vi "Ka-THWAP grabbers.vi"(10 "Action":enum16{"None", "Left", "Right", "Yes"}(ring), 11 "Enum":T1) -> ()   [LabVIEW 2014]
uses:
  TypeDefs/SRE Enum.ctl
  <vilib>/Rock Robotics/WPI/Solenoid/WPI_SolenoidChannel.ctl
  <vilib>/Rock Robotics/WPI/Solenoid/WPI_SolenoidValue.ctl
  <vilib>/Rock Robotics/WPI/Solenoid/WPI_SolenoidOpenDouble.vi
  <vilib>/Rock Robotics/WPI/Solenoid/WPI_SolenoidSetEnum.vi
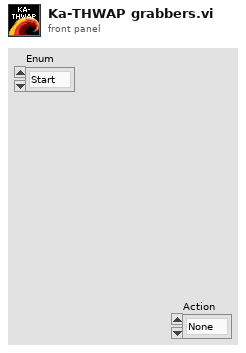
[diagram p1: front panel]
types:
  T1 = typedef "SRE Enum.ctl" = enum16{"Start", "Run", "End"}
  T2 = typedef "WPI_SolenoidChannel.ctl" = enum8{"Solenoid 0", "Solenoid 1", "Solenoid 2", "Solenoid 3", "Solenoid 4", "Solenoid 5", "Solenoid 6", "Solenoid 7", "Invalid"}
  T3 = typedef "WPI_SolenoidValue.ctl" = enum16{"Off", "On", "Forward", "Reverse"}
  T4 = typedef "WPI_SolenoidDevRef.ctl" = cluster{"DevStatus":errorcluster, "Pneumatics Control Module":u8, "Forward Solenoid Channel":T2, "Reverse Solenoid Channel":T2}
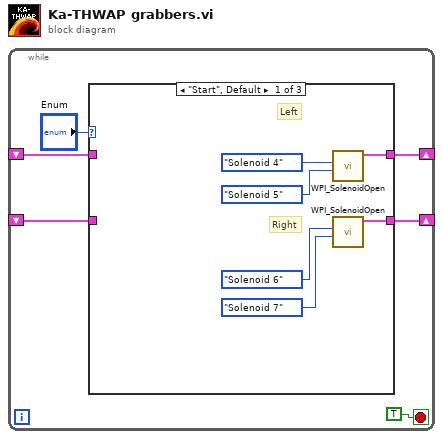
[diagram p0: block diagram]
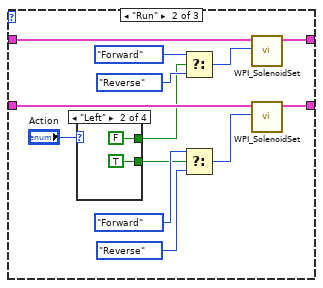
[diagram p2: hidden frame]
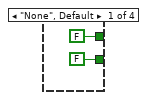
[diagram p3: hidden frame]
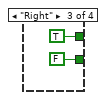
[diagram p4: hidden frame]
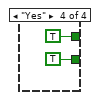
[diagram p5: hidden frame]
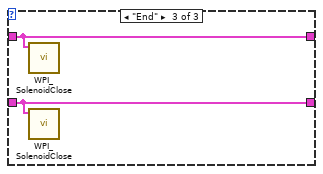
[diagram p6: hidden frame]
diagram:
  n1 = while {
    shift-right: [w4] -> _
    shift-left: _ -> [w2]
    shift-right: [w3] -> _
    shift-left: _ -> [w1]
    stop <- TRUE stop-if-true
    n2 = case shown="\"Start\", Default" "Enum" {
      tunnel: [w8 w18 w35] -> w4
      tunnel: [w7 w17 w34] -> w3
      tunnel: w2 -> [_ w19 w35]
      tunnel: w1 -> [_ w16 w34]
      frame "Start", Default {
        # "Right"
        # "Left"
        n3 = call-poly <vilib>:"WPI_SolenoidOpen.vi"("Reverse Solenoid Channel"=WPI_SolenoidChannel."Solenoid 5", "Forward Solenoid Channel"=WPI_SolenoidChannel."Solenoid 4" ("Solenoid Channel")) -> ("SolenoidDevRef"=w8:T4)  [unwired: 8 in, 1 out]
        n4 = call-poly <vilib>:"WPI_SolenoidOpen.vi"("Reverse Solenoid Channel"=WPI_SolenoidChannel."Solenoid 7", "Forward Solenoid Channel"=WPI_SolenoidChannel."Solenoid 6") -> ("SolenoidDevRef"=w7:T4)  [unwired: 8 in, 1 out]
      }
      frame "Run" {
        n5 = case shown="\"Left\"" "Action" {
          tunnel: [FALSE TRUE FALSE TRUE] -> w13
          tunnel: [FALSE FALSE TRUE TRUE] -> w14
          frame "None", Default {
          }
          frame "Left" {
          }
          frame "Right" {
          }
          frame "Yes" {
          }
        }
        n6 = Select(t=WPI_SolenoidValue."Forward" ("Value"), s=w14, f=WPI_SolenoidValue."Reverse") -> (s? t:f=w23:T3)
        n7 = Select(t=WPI_SolenoidValue."Forward" ("Value"), s=w13, f=WPI_SolenoidValue."Reverse") -> (s? t:f=w20:T3)
        n8 = call-poly <vilib>:"WPI_SolenoidSet.vi"("Value"=w23, "SolenoidDevRef"=w19) -> ("SolenoidDevRef"=w18:T4)  [unwired: 8 in, 1 out]
        n9 = call-poly <vilib>:"WPI_SolenoidSet.vi"("Value"=w20, "SolenoidDevRef"=w16) -> ("SolenoidDevRef"=w17:T4)  [unwired: 8 in, 1 out]
      }
      frame "End" {
        n10 = call <vilib>:"WPI_SolenoidClose.vi"("SolenoidDevRef"=w35) -> ()  [unwired: 10 in, 1 out]
        n11 = call <vilib>:"WPI_SolenoidClose.vi"("SolenoidDevRef"=w34) -> ()  [unwired: 10 in, 1 out]
      }
    }
  }
